vi "AddDependency.vi"(7 "Level":string, 8 "error in (no error)":errorcluster, 10 "Dependency":refnum<class "SMO.lvclass">, 11 "SMO in":refnum<class "SMO.lvclass">) -> (0 "error out":errorcluster, 2 "Unique Name":string, 3 "SMO out":refnum<class "SMO.lvclass">)   [LabVIEW 2021, in "smo.lvlib" / "SMO.lvclass"]
uses:
  SMO.lvclass
  Typedefs/SMO Dependency Event--Cluster.ctl
  Typedefs/SMO Dependency Event--Enum.ctl
  SMO.lvclass/SMO.ctl
  Support/Attribute.Identity/Attribute.Identity.lvclass/Attribute.Identity.ctl
  Support/Attribute.Identity/Read GUID.vi
  GetVariant(Attr).vi
  Support/Attribute.Identity/Read UniqueName.vi
  ReftoDVR--SMO.vi
  <vilib>/regexp/Match Regular Expression.xnode
  Support/Attribute.Identity/Attribute.Identity.lvclass
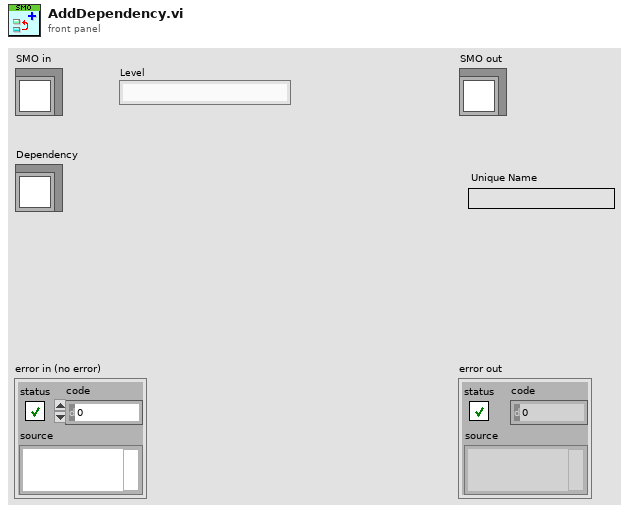
[diagram p1: front panel]
types:
  T1 = typedef "smo.lvlib/SMO.lvclass/SMO Dependency Event--Enum.ctl" = enum16{"Added", "Removed", "Started", "Stopped"}
  T2 = typedef "smo.lvlib/SMO.lvclass/SMO Dependency Event--Cluster.ctl" = cluster{"Name":string, "GUID":string, "Event":T1}
  T3 = typedef "smo.lvlib/SMO.lvclass/Protected Events.ctl" = cluster{"StopProcesses":refnum<user-event>, "AbortProcesses":refnum<user-event>, "Config Changed":refnum<user-event>, "Dependency":refnum<user-event>}
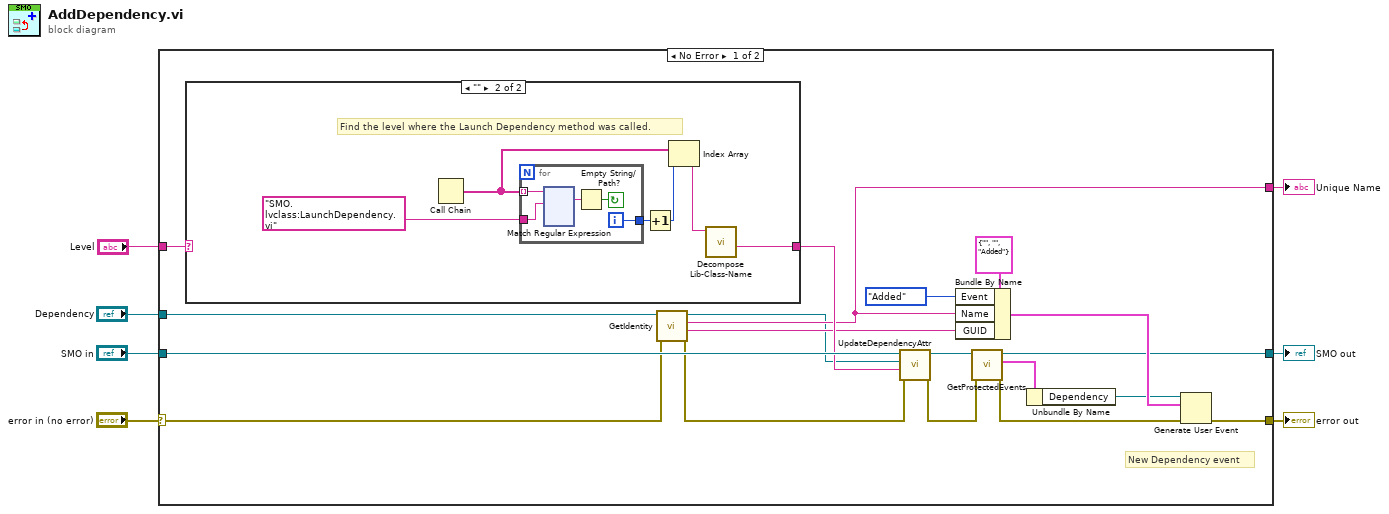
[diagram p0: block diagram]
diagram:
  n1 = case shown="No Error" "error in (no error)" {
    selector: "error in (no error)" -> [w8 w156]
    tunnel: "Level" -> [w26 _]
    tunnel: [w25 w156] -> w6
    tunnel: "SMO in" -> [w21 w157]
    tunnel: [w15 w157] -> w4
    tunnel: "Dependency" -> [w13 _]
    tunnel: [w12 _] -> w2
    frame No Error {
      # "New Dependency event"
      n2 = case shown="\"\"" w26 {
        selector: w26 -> [w27 _]
        tunnel: [w27 w28] -> w20
        frame Default {
        }
        frame "" {
          # "Find the level where the Launch Dependency method was called."
          n3 = Call Chain() -> (call chain=w33:string[])
          n4 = for {
            tunnel: w33 -> [w38] mode=indexing
            tunnel: "SMO.lvclass:LaunchDependency.vi" -> [w37]
            tunnel: [w34] -> w32
            i -> [w34]
            stop <- w35 continue-if-true
            n5 = xnode "Match Regular Expression"("input string"=w38, "regular expression"=w37) -> ("whole match"=w36:string)  [unwired: 4 in, 4 out]
            n6 = Empty String/Path?(string/path=w36) -> (empty?=w35:bool)
          }
          n7 = Increment(x=w32) -> (x+1=w31:i32)
          n8 = Index Array(array=w33, index=w31) -> (element=w29:string)
          n9 = call "Decompose Lib-Class-Name.vi"("Qualified Name"=w29) -> ("className"=w28:string)  [unwired: 6 in, 4 out]
        }
      }
      n10 = call "GetIdentity.vi"("error in (no error)"=w8, "SMO in"=w13) -> ("error out"=w9:errorcluster, "GUID"=w11:string, "Name"=w12:string, "SMO out"=w10:refnum<class "SMO.lvclass">)  [unwired: 6 in]
      n11 = call "UpdateDependencyAttr.vi"("error in (no error)"=w9, "Level"=w20, "Dependency"=w10, "SMO in"=w21) -> ("error out"=w16:errorcluster, "SMO out"=w19:refnum<class "SMO.lvclass">)  [unwired: 6 in]
      n12 = Bundle By Name(cluster=T2 {"Name"="", "GUID"="", "Event"=enum."Added"} ("Dependency Event"), "Event"=SMO_Dependency_Event--Enum."Added", "Name"=w12, "GUID"=w11) -> (w23:T2)
      n13 = call "GetProtectedEvents.vi"("error in (no error)"=w16, "SMO"=w19) -> ("error out"=w14:errorcluster, "SMO Protected Events"=w18:T3, "SMO out"=w15:refnum<class "SMO.lvclass">)  [unwired: 7 in]
      n14 = Unbundle By Name(w18) -> ("Dependency"=w17:refnum<user-event>)
      n15 = Generate User Event(user event=w17, event data cluster=w23, error in=w14) -> (error out=w25:errorcluster)  [unwired: 1 in, 1 out]
    }
    frame Error {
    }
  }
  "error out" <- w6
  "SMO out" <- w4
  "Unique Name" <- w2
